vi "CalpointMenu.vi"(8 "SYS|Plot|IDs":refnum<vi>, 9 "SYS|Plot|Units":refnum<vi>, 10 "SYS|Plot|Names":refnum<vi>, 11 "_QuickValues":refnum<vi>) -> ()   [LabVIEW 2016]
uses:
  Shared/Typedefs/System-QuickIDsArray.ctl
  <vilib>/addons/Software Calibration Management/xSCM/Controls/ID and Element.ctl
  <vilib>/Utility/miscctls.llb/LVRowAndColumnTypeDef.ctl
  <vilib>/addons/Software Calibration Management/xSCM/SCM-API.lvlib
  Shared/DSI-Shared.lvlib
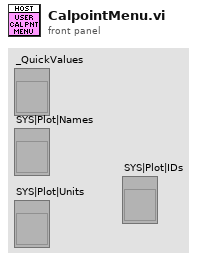
[diagram p1: front panel]
types:
  T1 = typedef "LVRowAndColumnTypeDef.ctl" = cluster{"Row":i32, "Column":i32}
  T2 = typedef "SCM-API.lvlib/ID and Element.ctl" = cluster{"ID":u32, "Element":i32[]}
  T3 = typedef "LVRowAndColumnUnsignedTypeDef.ctl" = cluster{"Row":u32, "Column":u32}
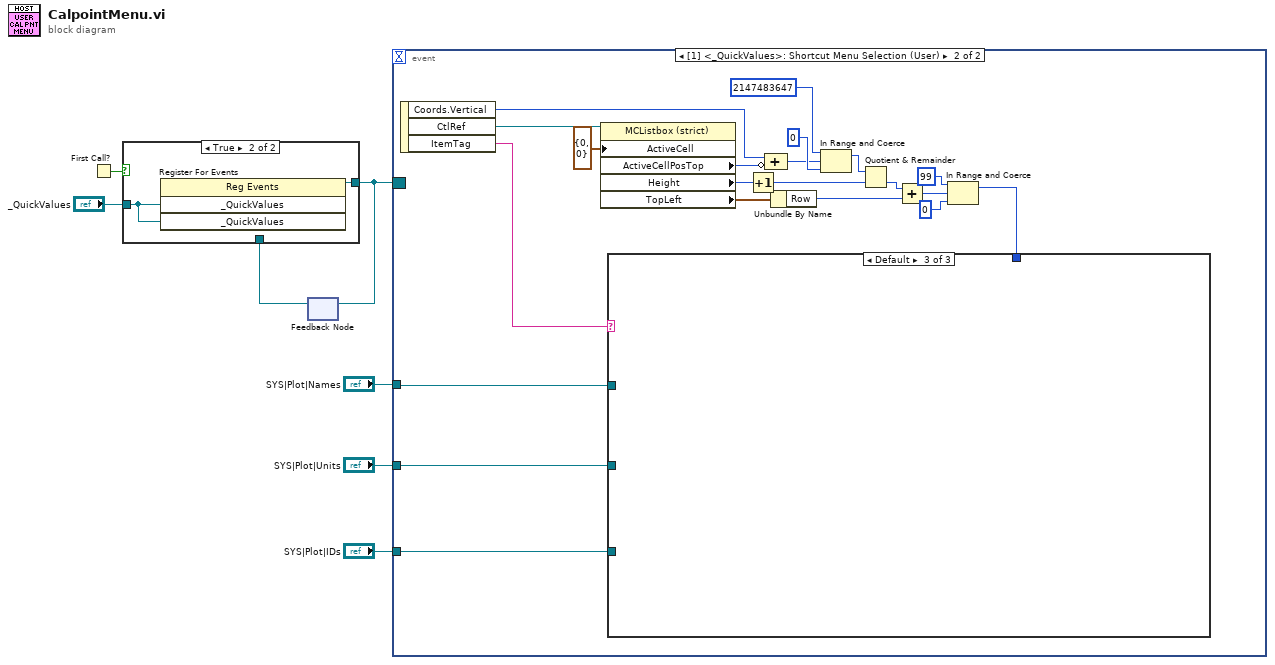
[diagram p0: block diagram]
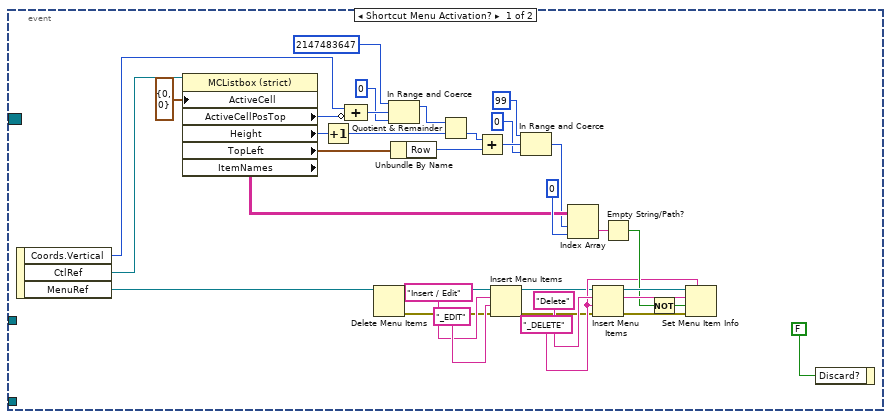
[diagram p2: hidden frame]
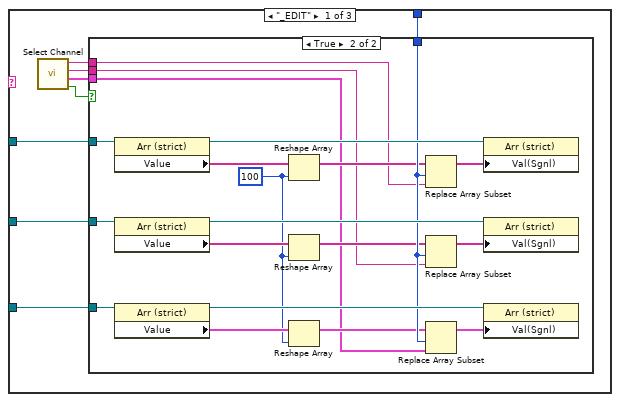
[diagram p3: hidden frame]
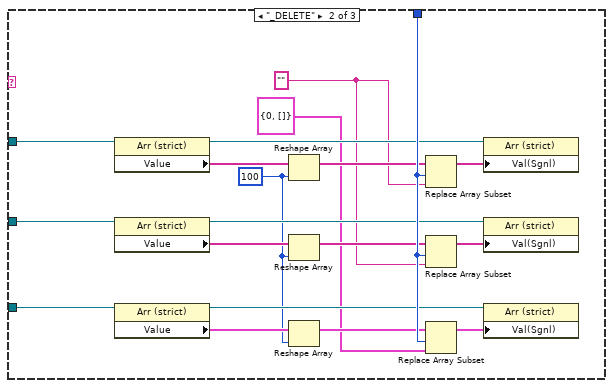
[diagram p5: hidden frame]
diagram:
  n1 = First Call?() -> (First Call?: T/F=w7:bool)
  n2 = feedback #1() -> (w5:refnum<event-registration>)  [unwired: 1 in]
  n3 = case shown="True" w7 {
    tunnel: "_QuickValues" -> [_ w10]
    tunnel: [w8 w9] -> w6
    tunnel: w5 -> [w8 _]
    frame False {
    }
    frame True {
      n4 = register-events(w10, w10) -> (reference out=w9:refnum<event-registration>)  [unwired: 2 in, 1 out]
    }
  }
  n5 = feedback-in #1(w6) -> ()
  n6 = event shown="[1] <_QuickValues>: Shortcut Menu Selection (User)" {
    selector: w6 -> [_ _]
    dyn-events: _ -> [_ _]
    timeout: _ -> [_ _]
    tunnel: "SYS|Plot|Names" -> [_ w47]
    tunnel: "SYS|Plot|Units" -> [_ w46]
    tunnel: "SYS|Plot|IDs" -> [_ w45]
    event Shortcut Menu Activation? {
      w42 = "Delete" ("item names")
      w31 = "_DELETE" ("format string")
      n7 = event-data() -> ("Coords.Vertical"=w21:i32, "CtlRef"=w34:refnum<vi>, "MenuRef"=w44:refnum<k9>)  [unwired: 1 in]
      n8 = property on="Property Node" class="MCListbox (strict)"(reference=w34, "ActiveCell"=T1 {"Row"=0, "Column"=0} ("Active Cell:Active Cell")) -> ("ActiveCellPosTop"=w22:i32, "Height"=w37:u32, "TopLeft"=w36:T3, "ItemNames"=w38:string[][])  [unwired: 1 in, 2 out]
      n9 = Increment(x=w37) -> (x+1=w19:u32)
      n10 = Compound Arithmetic op=ADD(w21, invert w22) -> (w15:i32)
      n11 = Delete Menu Items(9:w44) -> (0:w27:errorcluster, 3:w28:refnum<k9>)  [unwired: 3 in]
      n12 = In Range and Coerce(upper limit=2147483647, x=w15, lower limit=0) -> (coerced(x)=w12:i32)  [unwired: 1 out]
      n13 = Unbundle By Name(w36) -> ("Row"=w35:u32)
      n14 = Quotient & Remainder(x=w12, y=w19) -> (floor(x/y)=w11:u32)  [unwired: 1 out]
      n15 = Add(x=w11, y=w35) -> (x+y=w20:u32)
      n16 = Insert Menu Items(6:w27, 7:"_EDIT" ("format string"), 8:"Insert / Edit" ("item names"), 9:w28) -> (0:w26:errorcluster, 3:w25:refnum<k9>)  [unwired: 2 in, 1 out]
      n17 = In Range and Coerce(upper limit=u32 99, x=w20, lower limit=u32 0) -> (coerced(x)=w18:u32)  [unwired: 1 out]
      n18 = Index Array(array=w38, index (row)=w18, index (col)=0 ("disabled index (col)")) -> (element=w40:string)
      n19 = Insert Menu Items(6:w26, 7:w31, 8:w42, 9:w25) -> (0:w41:errorcluster, 3:w43:refnum<k9>)  [unwired: 2 in, 1 out]
      n20 = Empty String/Path?(string/path=w40) -> (empty?=w33:bool)
      n21 = Not(x=w33) -> (.not. x?=w32:bool)
      n22 = Set Menu Item Info(7:w31, 8:w41, 9:w32, 10:w42, 11:w43) -> ()  [unwired: 2 in, 2 out]
      n23 = event-data("Discard?"=FALSE) -> ()  [unwired: 1 in, 1 out]
    }
    event Shortcut Menu Selection (User) {
      n24 = event-data() -> ("Coords.Vertical"=w64:i32, "CtlRef"=w65:refnum<vi>, "ItemTag"=w49:string)  [unwired: 1 in]
      n25 = property on="Property Node" class="MCListbox (strict)"(reference=w65, "ActiveCell"=T1 {"Row"=0, "Column"=0} ("Active Cell:Active Cell")) -> ("ActiveCellPosTop"=w63:i32, "Height"=w62:u32, "TopLeft"=w61:T3)  [unwired: 1 in, 2 out]
      n26 = Increment(x=w62) -> (x+1=w57:u32)
      n27 = Compound Arithmetic op=ADD(w64, invert w63) -> (w51:i32)
      n28 = Unbundle By Name(w61) -> ("Row"=w59:u32)
      n29 = In Range and Coerce(upper limit=2147483647, x=w51, lower limit=0) -> (coerced(x)=w50:i32)  [unwired: 1 out]
      n30 = Quotient & Remainder(x=w50, y=w57) -> (floor(x/y)=w60:u32)  [unwired: 1 out]
      n31 = Add(x=w60, y=w59) -> (x+y=w54:u32)
      n32 = In Range and Coerce(upper limit=u32 99, x=w54, lower limit=u32 0) -> (coerced(x)=w48:u32)  [unwired: 1 out]
      n33 = case shown="Default" w49 {
        tunnel: w48 -> [w70 w112 _]
        tunnel: w47 -> [w68 w111 _]
        tunnel: w46 -> [w67 w110 _]
        tunnel: w45 -> [w66 w109 _]
        frame "_EDIT" {
          n34 = call <vilib>:"Select Channel.vi"() -> ("OK"=w69:bool, "ID"=w73:T2, "Units"=w72:string, "Name"=w71:string)  [unwired: 8 in]
          n35 = case shown="True" w69 {
            tunnel: w66 -> [_ w91]
            tunnel: w68 -> [_ w90]
            tunnel: w67 -> [_ w88]
            tunnel: w70 -> [_ w81]
            tunnel: w73 -> [_ w76]
            tunnel: w72 -> [_ w75]
            tunnel: w71 -> [_ w74]
            frame False {
            }
            frame True {
              w77 = 100 ("dimension size")
              n36 = property on="Property Node" class="Arr (strict)"(reference=w90) -> (reference out=w89:refnum<vi>, "Value"=w85:string[])  [unwired: 1 in, 1 out]
              n37 = property on="Property Node" class="Arr (strict)"(reference=w88) -> (reference out=w87:refnum<vi>, "Value"=w86:string[])  [unwired: 1 in, 1 out]
              n38 = property on="Property Node" class="Arr (strict)"(reference=w91) -> (reference out=w84:refnum<vi>, "Value"=w82:T2[])  [unwired: 1 in, 1 out]
              n39 = Reshape Array(w85, w77) -> (w78:string[])
              n40 = Reshape Array(w86, w77) -> (w79:string[])
              n41 = Reshape Array(w82, w77) -> (w80:T2[])
              n42 = Replace Array Subset(array=w78, new element=w74, index=w81) -> (w92:string[])
              n43 = Replace Array Subset(array=w79, new element=w75, index=w81) -> (w93:string[])
              n44 = Replace Array Subset(array=w80, new element=w76, index=w81) -> (w83:T2[])
              n45 = property on="Property Node" class="Arr (strict)"(reference=w89, "Val(Sgnl)"=w92) -> ()  [unwired: 1 in, 2 out]
              n46 = property on="Property Node" class="Arr (strict)"(reference=w87, "Val(Sgnl)"=w93) -> ()  [unwired: 1 in, 2 out]
              n47 = property on="Property Node" class="Arr (strict)"(reference=w84, "Val(Sgnl)"=w83) -> ()  [unwired: 1 in, 2 out]
            }
          }
        }
        frame "_DELETE" {
          w95 = "" ("Units")
          w96 = 100 ("dimension size")
          n48 = property on="Property Node" class="Arr (strict)"(reference=w111) -> (reference out=w106:refnum<vi>, "Value"=w103:string[])  [unwired: 1 in, 1 out]
          n49 = property on="Property Node" class="Arr (strict)"(reference=w110) -> (reference out=w105:refnum<vi>, "Value"=w104:string[])  [unwired: 1 in, 1 out]
          n50 = property on="Property Node" class="Arr (strict)"(reference=w109) -> (reference out=w102:refnum<vi>, "Value"=w100:T2[])  [unwired: 1 in, 1 out]
          n51 = Reshape Array(w103, w96) -> (w97:string[])
          n52 = Reshape Array(w104, w96) -> (w98:string[])
          n53 = Reshape Array(w100, w96) -> (w99:T2[])
          n54 = Replace Array Subset(array=w97, new element=w95, index=w112) -> (w107:string[])
          n55 = Replace Array Subset(array=w98, new element=w95, index=w112) -> (w108:string[])
          n56 = Replace Array Subset(array=w99, new element=T2 {"ID"=0, "Element"=[]} ("ID"), index=w112) -> (w101:T2[])
          n57 = property on="Property Node" class="Arr (strict)"(reference=w106, "Val(Sgnl)"=w107) -> ()  [unwired: 1 in, 2 out]
          n58 = property on="Property Node" class="Arr (strict)"(reference=w105, "Val(Sgnl)"=w108) -> ()  [unwired: 1 in, 2 out]
          n59 = property on="Property Node" class="Arr (strict)"(reference=w102, "Val(Sgnl)"=w101) -> ()  [unwired: 1 in, 2 out]
        }
        frame Default {
        }
      }
    }
  }
